vi "SEC Main.vi"() -> ()   [LabVIEW 2009]
doc: "This is the Main VI for the Security System application. The Security System application monitors Alarm Switches and reports Zone Status information. Alarms can be Bypassed. Alarms also have Tamper Switches."
uses:
  controls/sec_AlarmControls_cluster.ctl
  controls/sec_AlarmStatus_cluster.ctl
  controls/sec_ConsumerDataType_cluster.ctl
  controls/sec_ConsumerCommand_enum.ctl
  modules/error/sec_Error_Command_enum.ctl
  modules/alarm logging/sec_Log_Command_enum.ctl
  modules/alarm colors/sec_AlarmColors_Command_enum.ctl
  modules/alarms/sec_AlarmLogic_Command_enum.ctl
panel:
  out "error out":errorcluster
  in  "error in (no error)":errorcluster
  in  "Stop":bool
  in  "Tamper Switches":T1
  in  "Bypass Switches":T1
  out "Zone Status Indicators":T2
  in  "Alarm Switches":T1
  # "Green = Normal\nRed = Alarm\nOrange = Tamper\nBlue = Bypass"
  # "1"
  # "2"
  # "3"
  # "4"
  # "5"
  # "6"
  # "Zone"
  # "Alarm Switches"
  # "Bypass Switches"
  # "Tamper Switches"
  # "Zone Status Indicators"
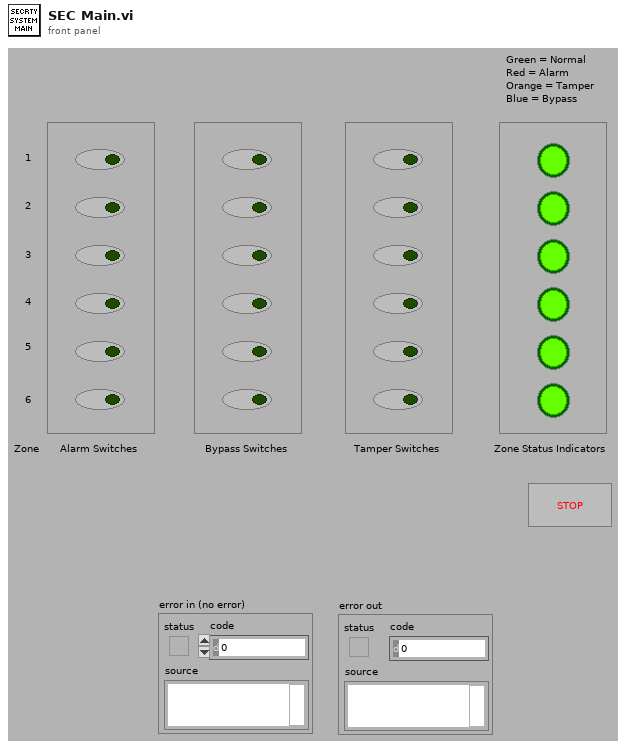
[diagram p1: front panel]
types:
  T1 = typedef "sec_AlarmControls_cluster.ctl" = cluster{"Boolean":bool, "Boolean 2":bool, "Boolean 3":bool, "Boolean 4":bool, "Boolean 5":bool, "Boolean 6":bool}
  T2 = typedef "sec_AlarmStatus_cluster.ctl" = cluster{"Boolean":bool, "Boolean 2":bool, "Boolean 3":bool, "Boolean 4":bool, "Boolean 5":bool, "Boolean 6":bool}
  T3 = typedef "sec_Error_Command_enum.ctl" = enum16{"Initialise", "Check Error", "Report Errors"}
  T4 = typedef "sec_ConsumerDataType_cluster.ctl" = cluster{"Command":T5, "Data":variant}
  T5 = typedef "sec_ConsumerCommand_enum.ctl" = enum16{"Initialise", "Get Front Panel Data", "Set Front Panel Data", "Switch Updated", "Shutdown"}
  T6 = typedef "sec_Log_Command_enum.ctl" = enum16{"Initialise", "Log Alarms"}
  T7 = typedef "sec_AlarmColors_Command_enum.ctl" = enum16{"Initialise", "Set Alarm States", "Update Alarm Status Display", "Shutdown"}
  T8 = typedef "sec_AlarmLogic_Command_enum.ctl" = enum16{"Initialise", "Set Alarm Switches", "Check Alarm States", "Get Alarm States"}
  T9 = cluster{"Alarm Status[0]":bool, "Alarm Status[1]":bool, "Alarm Status[2]":bool, "Alarm Status[3]":bool, "Alarm Status[4]":bool, "Alarm Status[5]":bool}
  T10 = typedef "sec_AlarmStates_enum.ctl" = enum16{"Normal", "Alarm", "Bypass", "Tamper"}
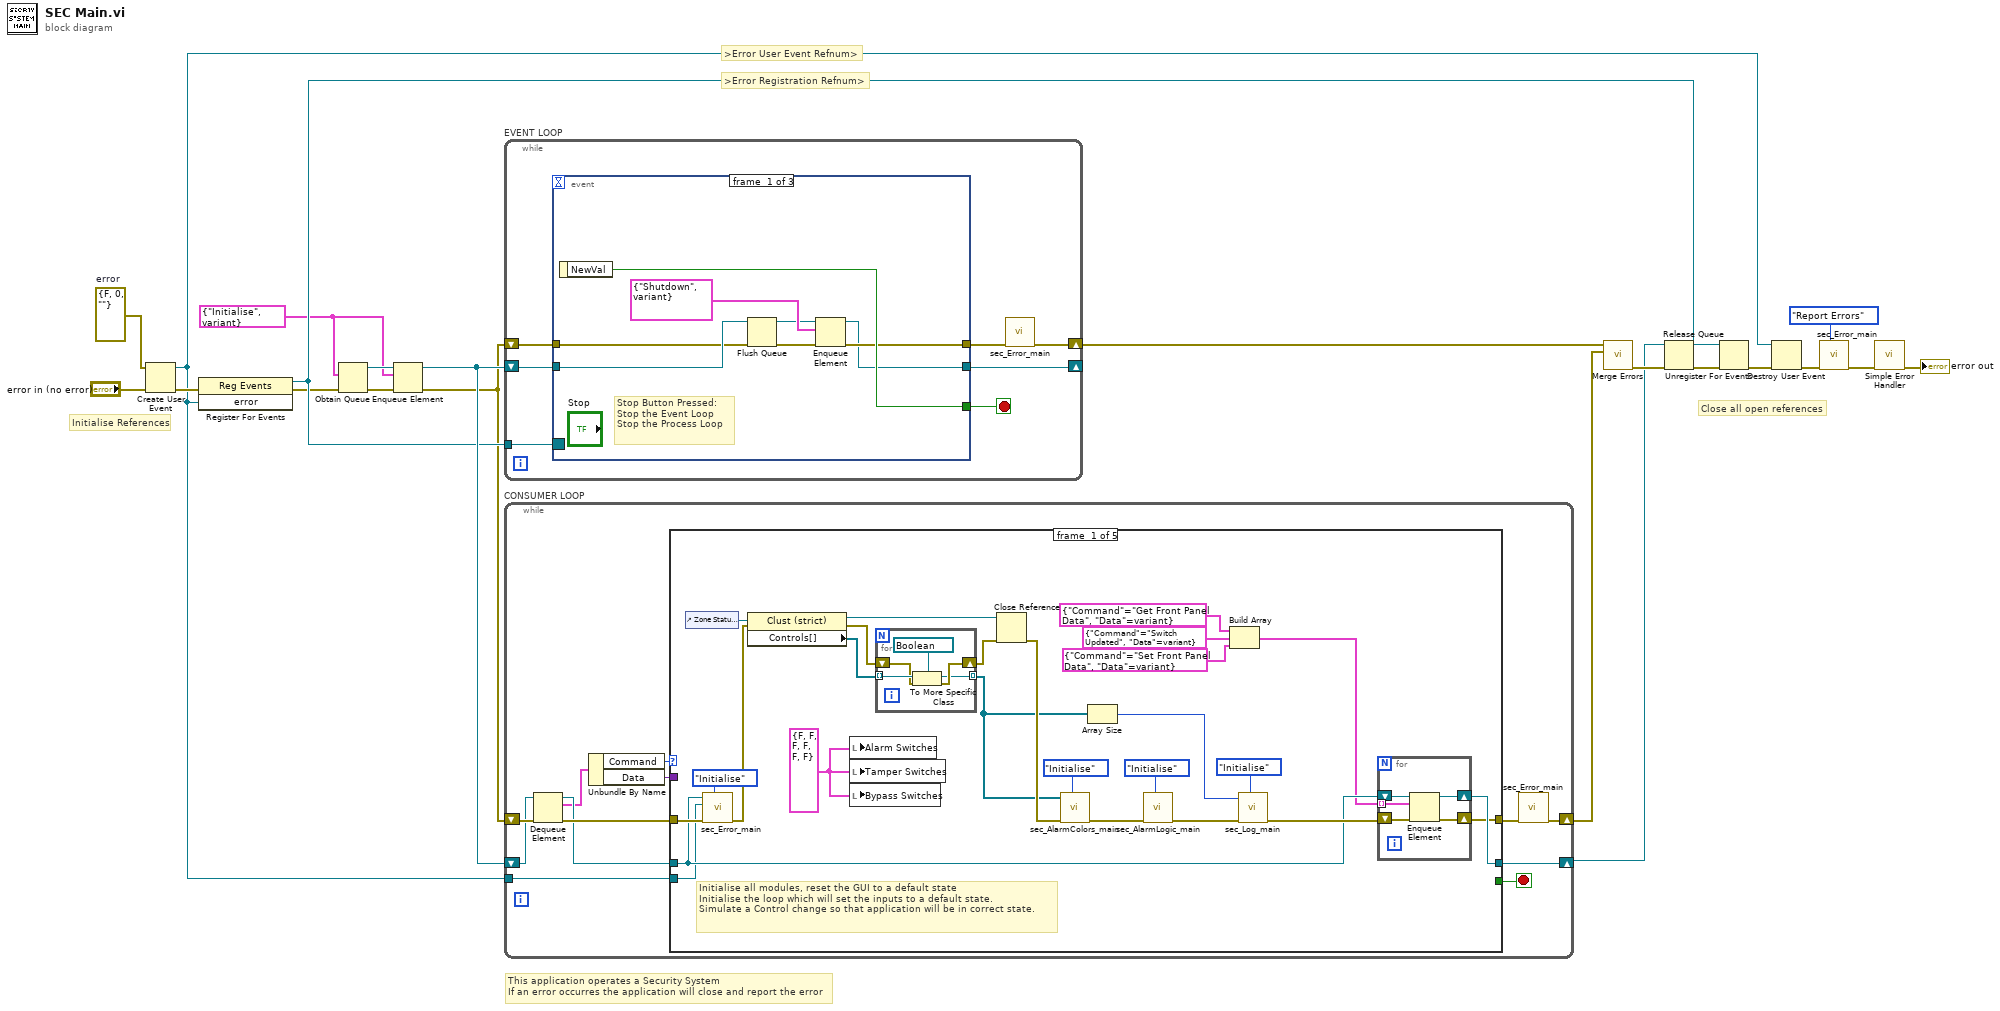
[diagram p0: block diagram]
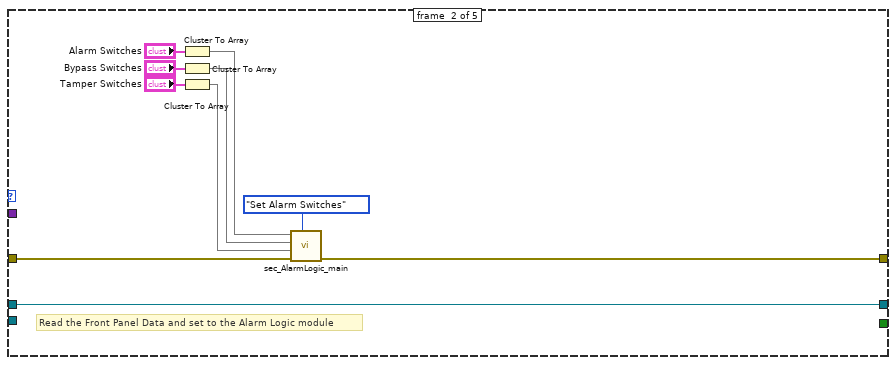
[diagram p2: hidden frame]
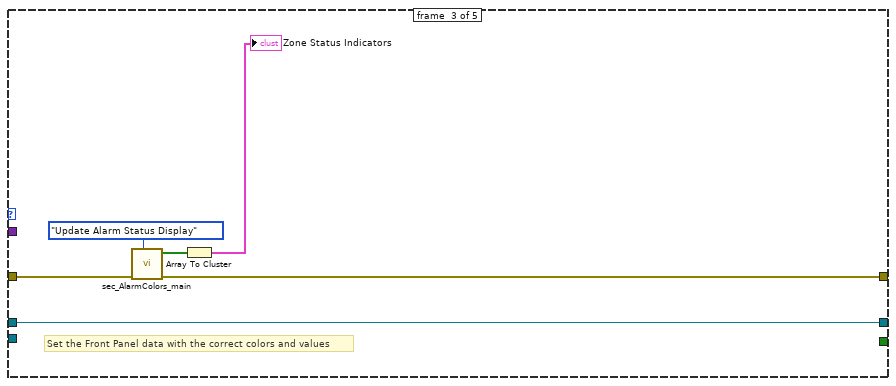
[diagram p3: hidden frame]
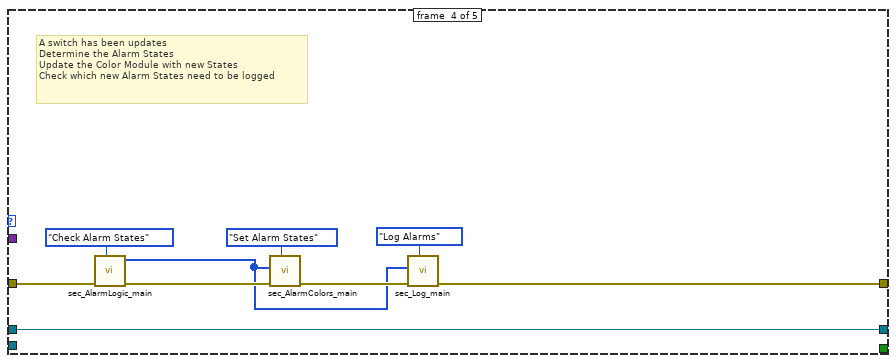
[diagram p4: hidden frame]
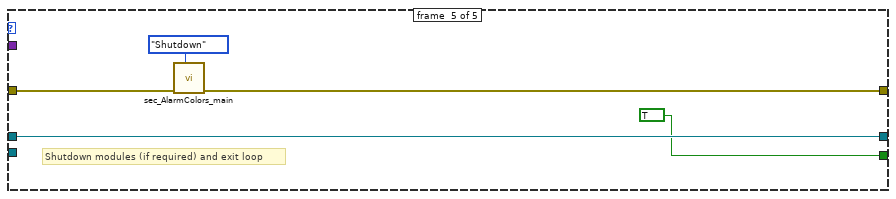
[diagram p5: hidden frame]
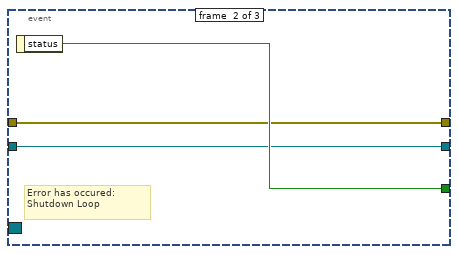
[diagram p6: hidden frame]
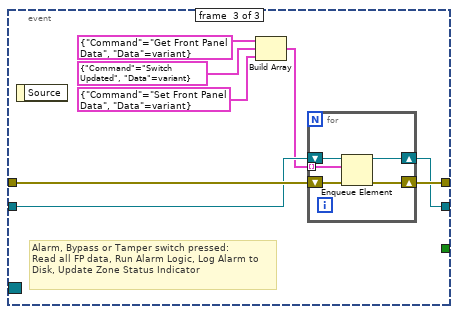
[diagram p7: hidden frame]
diagram:
  w7 = errorcluster {"status"=FALSE, "code"=0, "source"=""}  # error
  w2 = T4 {"Command"=enum."Initialise", "Data"=variant} ("State Data")
  # ">Error Registration Refnum>"
  # ">Error User Event Refnum>"
  # "Initialise References"
  # "Close all open references"
  # "This application operates a Security System\nIf an error occurres the application will close and report the error"
  n1 = Create User Event(user event datatype=w7, error in="error in (no error)") -> (user event=w15:refnum<user-event>, error out=w17:errorcluster)
  n2 = register-events(error in=w17, w15) -> (reference out=w16:refnum<event-registration>, error out=w5:errorcluster)  [unwired: 1 in]
  n3 = Obtain Queue(element data type=w2, error in (no error)=w5) -> (queue out=w20:refnum<queue>, error out=w21:errorcluster)  [unwired: 3 in, 1 out]
  n4 = Enqueue Element(queue=w20, element=w2, error in (no error)=w21) -> (queue out=w18:refnum<queue>, error out=w4:errorcluster)  [unwired: 1 in, 1 out]
  n5 = while "EVENT LOOP" {
    shift-right: [w23] -> w13
    shift-left: w4 -> [w27]
    shift-right: [w25] -> _
    shift-left: w18 -> [w26]
    tunnel: w16 -> [w24]
    stop <- w28 stop-if-true
    n6 = event shown="[1] <error>: User Event" {
      selector: w24 -> [_ _ _]
      dyn-events: _ -> [_ _ _]
      timeout: _ -> [_ _ _]
      tunnel: [w36 w39 _] -> w28
      tunnel: w27 -> [w30 w37 w47]
      tunnel: [w35 w37 w46] -> w22
      tunnel: w26 -> [w32 w38 w45]
      tunnel: [w34 w38 w44] -> w25
      event #0 {
        # "Stop Button Pressed:\nStop the Event Loop\nStop the Process Loop"
        n7 = event-data() -> ("NewVal"=w36:bool)  [unwired: 1 in]
        n8 = Flush Queue(queue=w32, error in (no error)=w30) -> (queue out=w31:refnum<queue>, error out=w29:errorcluster)  [unwired: 1 out]
        n9 = Enqueue Element(queue=w31, element=T4 {"Command"=enum."Shutdown", "Data"=variant} ("State Data"), error in (no error)=w29) -> (queue out=w34:refnum<queue>, error out=w35:errorcluster)  [unwired: 1 in, 1 out]
      }
      event #1 {
        # "Error has occured:\nShutdown Loop"
        n10 = event-data() -> ("status"=w39:bool)  [unwired: 1 in]
      }
      event #2 {
        # "Alarm, Bypass or Tamper switch pressed: \nRead all FP data, Run Alarm Logic, Log Alarm to Disk, Update Zone Status Indicator"
        n11 = event-data() -> ()  [unwired: 1 in, 1 out]
        n12 = Build Array(T4 {"Command"=enum."Get Front Panel Data", "Data"=variant} ("State Data"), T4 {"Command"=enum."Switch Updated", "Data"=variant} ("State Data"), T4 {"Command"=enum."Set Front Panel Data", "Data"=variant} ("State Data")) -> (w40:T4[])
        n13 = for {
          tunnel: w40 -> [w48] mode=indexing
          shift-right: [w49] -> w44
          shift-left: w45 -> [w50]
          shift-right: [w51] -> w46
          shift-left: w47 -> [w52]
          n14 = Enqueue Element(queue=w50, element=w48, error in (no error)=w52) -> (queue out=w49:refnum<queue>, error out=w51:errorcluster)  [unwired: 1 in, 1 out]
        }
      }
    }
    n15 = call "sec_Error_main.vi"("error in (no error)"=w22) -> ("error out"=w23:errorcluster)  [unwired: 10 in]
  }
  n16 = while "CONSUMER LOOP" {
    shift-right: [w55] -> w19
    shift-left: w4 -> [w64]
    shift-right: [w53] -> w3
    shift-left: w18 -> [w61]
    tunnel: w15 -> [w56]
    stop <- w58 stop-if-true
    n17 = Dequeue Element(queue=w61, error in (no error)=w64) -> (queue out=w62:refnum<queue>, element=w60:T4, error out=w63:errorcluster)  [unwired: 1 in, 1 out]
    n18 = Unbundle By Name(w60) -> ("Command"=w57:T5, "Data"=w59:variant)
    n19 = case shown="\"Initialise\", Default" w57 {
      tunnel: w63 -> [w76 w106 w114 w124 w126]
      tunnel: w62 -> [w72 w110 w116 w125 w130]
      tunnel: [w71 w110 w116 w125 w130] -> w53
      tunnel: [w65 w105 w113 w117 w127] -> w54
      tunnel: w59 -> [_ _ _ _ _]
      tunnel: [_ _ _ _ TRUE] -> w58
      tunnel: w56 -> [w66 _ _ _ _]
      frame #0 {
        w81 = T1 {"Boolean"=FALSE, "Boolean 2"=FALSE, "Boolean 3"=FALSE, "Boolean 4"=FALSE, "Boolean 5"=FALSE, "Boolean 6"=FALSE} ("Tamper Switches")
        # "Initialise all modules, reset the GUI to a default state\nInitialise the loop which will set the inputs to a default state. \nSimulate a Control change so that application will be in correct state."
        n20 = control-ref of="Zone Status Indicators"() -> (w88:refnum<vi>)
        n21 = call "sec_Error_main.vi"("Command (Check Error)"=sec_Error_Command_enum."Initialise", "error in (no error)"=w76, "Error Event Refnum"=w66, "Process Loop Queue Refnum"=w72) -> ("error out"=w75:errorcluster)  [unwired: 7 in]
        n22 = property class="Clust (strict)"(reference=w88, error in=w75) -> (reference out=w84:refnum<vi>, error out=w86:errorcluster, "Controls[]"=w87:refnum<vi>[])
        n23 = local write "Alarm Switches"(w81) -> ()
        n24 = local write "Tamper Switches"(w81) -> ()
        n25 = local write "Bypass Switches"(w81) -> ()
        n26 = for {
          tunnel: w87 -> [w100] mode=indexing
          shift-right: [w98] -> w85
          shift-left: w86 -> [w99]
          tunnel: [w96] -> w78 mode=indexing
          n27 = To More Specific Class(target class=refnum<vi> refnum ("specific class reference"), reference=w100, error in=w99) -> (specific class reference=w96:refnum<vi>, error out=w98:errorcluster)
        }
        n28 = Close Reference(reference=w84, error in (no error)=w85) -> (error out=w83:errorcluster)
        n29 = call "sec_AlarmColors_main.vi"("Command"=sec_AlarmColors_Command_enum."Initialise", "error in (no error)"=w83, "Status Zone Refnums"=w78) -> ("error out"=w82:errorcluster)  [unwired: 7 in, 1 out]
        n30 = Array Size(array=w78) -> (size(s)=w77:i32)
        n31 = call "sec_AlarmLogic_main.vi"("Command"=sec_AlarmLogic_Command_enum."Initialise", "error in (no error)"=w82) -> ("error out"=w79:errorcluster)  [unwired: 8 in, 1 out]
        n32 = Build Array(T4 {"Command"=enum."Get Front Panel Data", "Data"=variant} ("State Data"), T4 {"Command"=enum."Switch Updated", "Data"=variant} ("State Data"), T4 {"Command"=enum."Set Front Panel Data", "Data"=variant} ("State Data")) -> (w67:T4[])
        n33 = call "sec_Log_main.vi"("Command"=sec_Log_Command_enum."Initialise", "error in (no error)"=w79, "Number Of Alarms"=w77) -> ("error out"=w73:errorcluster)  [unwired: 8 in]
        n34 = for {
          shift-right: [w92] -> w71
          shift-left: w72 -> [w93]
          shift-right: [w94] -> w65
          shift-left: w73 -> [w95]
          tunnel: w67 -> [w91] mode=indexing
          n35 = Enqueue Element(queue=w93, element=w91, error in (no error)=w95) -> (queue out=w92:refnum<queue>, error out=w94:errorcluster)  [unwired: 1 in, 1 out]
        }
      }
      frame #1 {
        # "Read the Front Panel Data and set to the Alarm Logic module"
        n36 = Cluster To Array(cluster="Alarm Switches") -> (array=w102:bool[])
        n37 = Cluster To Array(cluster="Bypass Switches") -> (array=w103:bool[])
        n38 = Cluster To Array(cluster="Tamper Switches") -> (array=w104:bool[])
        n39 = call "sec_AlarmLogic_main.vi"("Command"=sec_AlarmLogic_Command_enum."Set Alarm Switches", "error in (no error)"=w106, "Tamper Switches"=w104, "Bypass Switches"=w103, "Alarm Switches"=w102) -> ("error out"=w105:errorcluster)  [unwired: 5 in, 1 out]
      }
      frame #2 {
        # "Set the Front Panel data with the correct colors and values"
        n40 = call "sec_AlarmColors_main.vi"("Command"=sec_AlarmColors_Command_enum."Update Alarm Status Display", "error in (no error)"=w114) -> ("error out"=w113:errorcluster, "Alarm Status"=w111:bool[])  [unwired: 8 in]
        n41 = Array To Cluster(array=w111) -> (cluster=→"Zone Status Indicators":T9)
      }
      frame #3 {
        # "A switch has been updates\nDetermine the Alarm States \nUpdate the Color Module with new States\nCheck which new Alarm States need to be logged"
        n42 = call "sec_AlarmLogic_main.vi"("Command"=sec_AlarmLogic_Command_enum."Check Alarm States", "error in (no error)"=w124) -> ("error out"=w123:errorcluster, "Alarm States"=w118:T10[])  [unwired: 8 in]
        n43 = call "sec_AlarmColors_main.vi"("Command"=sec_AlarmColors_Command_enum."Set Alarm States", "error in (no error)"=w123, "Alarm States"=w118) -> ("error out"=w120:errorcluster)  [unwired: 7 in, 1 out]
        n44 = call "sec_Log_main.vi"("Command"=sec_Log_Command_enum."Log Alarms", "error in (no error)"=w120, "Alarm States"=w118) -> ("error out"=w117:errorcluster)  [unwired: 8 in]
      }
      frame #4 {
        # "Shutdown modules (if required) and exit loop"
        n45 = call "sec_AlarmColors_main.vi"("Command"=sec_AlarmColors_Command_enum."Shutdown", "error in (no error)"=w126) -> ("error out"=w127:errorcluster)  [unwired: 8 in, 1 out]
      }
    }
    n46 = call "sec_Error_main.vi"("error in (no error)"=w54) -> ("error out"=w55:errorcluster)  [unwired: 10 in]
  }
  n47 = call <vilib>:"Merge Errors.vi"("error in 2 (no error)"=w19, "error in 1 (no error)"=w13) -> ("error out"=w9:errorcluster)  [unwired: 5 in]
  n48 = Release Queue(queue=w3, error in (no error)=w9) -> (error out=w8:errorcluster)  [unwired: 1 in, 2 out]
  n49 = Unregister For Events(event registration refnum=w16, error in=w8) -> (error out=w14:errorcluster)
  n50 = Destroy User Event(user event=w15, error in=w14) -> (error out=w10:errorcluster)
  n51 = call "sec_Error_main.vi"("Command (Check Error)"=sec_Error_Command_enum."Report Errors", "error in (no error)"=w10) -> ("error out"=w12:errorcluster)  [unwired: 9 in]
  n52 = call <vilib>:"Simple Error Handler.vi"("error in (no error)"=w12) -> ("error out"=→"error out":errorcluster)  [unwired: 4 in, 4 out]
